vi "Initialize Front Panel controls.vi"(10 "Command":refnum<vi>, 11 "ListBox in":refnum<vi>) -> (0 "error out":errorcluster, 2 "Item Names":string[](array[string]), 3 "String out":refnum<vi>)   [LabVIEW 2013]
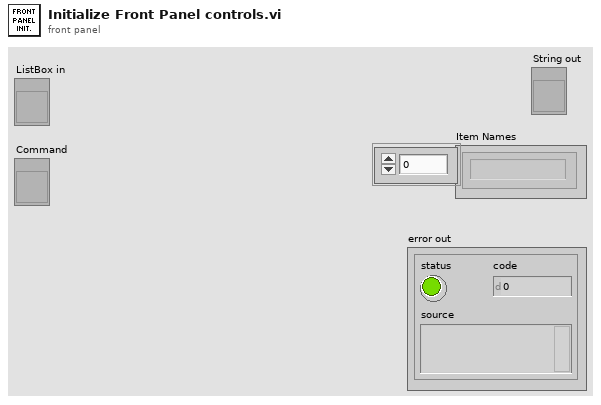
[diagram p1: front panel]
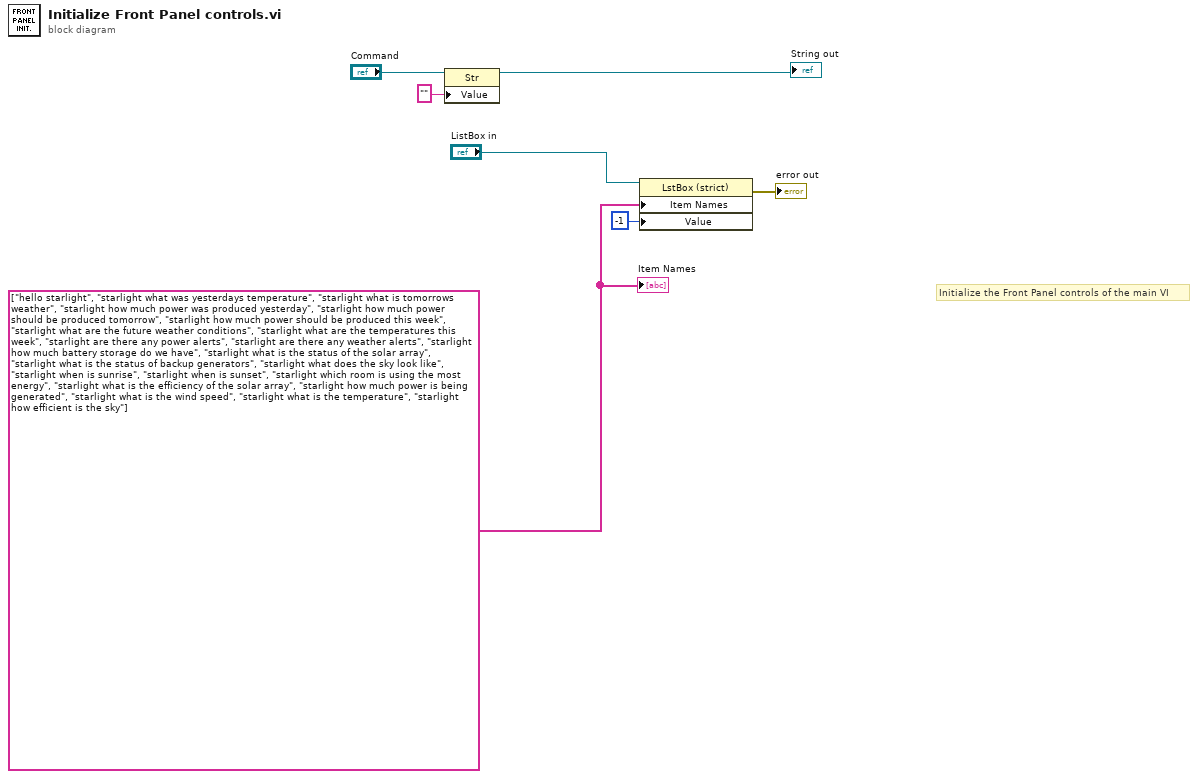
[diagram p0: block diagram]
diagram:
  w2 = string[] ["hello starlight", "starlight what was yesterdays temperature", "starlight what is tomorrows weather", "starlight how much power was produced yesterday", "starlight how much power should be produced tomorrow", "starlight how much power should be produced this week", "starlight what are the future weather conditions", "starlight what are the temperatures this week", "starlight are there any power alerts", "starlight are there any weather alerts", "starlight how much battery storage do we have", "starlight what is the status of the solar array", "starlight what is the status of backup generators", "starlight what does the sky look like", "starlight when is sunrise", "starlight when is sunset", "starlight which room is using the most energy", "starlight what is the efficiency of the solar array", "starlight how much power is being generated", "starlight what is the wind speed", "starlight what is the temperature", "starlight how efficient is the sky"] ("Item Names")
  # "Initialize the Front Panel controls of the main VI"
  n1 = property class="Str"(reference="Command", "Value"="") -> (reference out=→"String out":refnum<vi>)  [unwired: 1 in, 1 out]
  n2 = property on="Property Node" class="LstBox (strict)"(reference="ListBox in", "Item Names"=w2, "Value"=-1) -> (error out=→"error out":errorcluster)  [unwired: 1 in, 1 out]
  "Item Names" <- w2
